vi "Stop task.vi"(8 "error in":errorcluster, 10 "Task list":T1(ring), 11 "Module ID":i32=-1) -> (0 "error out":errorcluster)   [LabVIEW 2020, in "NI DAQ.lvlib"]
doc: "Request to stop all channels within the local task.\n_____\nCreated using DQMH Event Scripter 6.1.0.128."
uses:
  NI DAQ.lvlib
  Stop task Argument--cluster.ctl
  Support/Task list.ctl
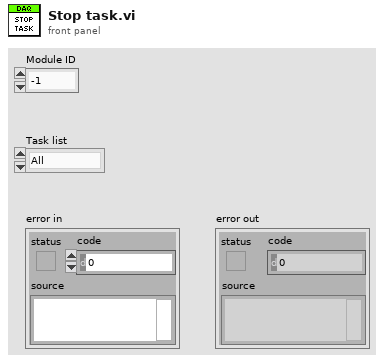
[diagram p1: front panel]
types:
  T1 = enum16{"All", "DO task", "DI task", "AO task", "AI task"}
  T2 = typedef "NI DAQ.lvlib/Stop task Argument--cluster.ctl" = cluster{"Module ID":i32, "Task list":T3}
  T3 = typedef "NI DAQ.lvlib/Task list.ctl" = enum16{"All", "DO task", "DI task", "AO task", "AI task"}
  T4 = typedef "NI DAQ.lvlib/Request Events--cluster.ctl" = cluster{"Stop Module":refnum<user-event>, "Show Panel":refnum<user-event>, "Hide Panel":refnum<user-event>, "Show Diagram":refnum<user-event>, "Get Module Execution Status":refnum<user-event>, "Set device ID":refnum<user-event>, "Get channel list":refnum<user-event>, "Create DO task":refnum<user-event>, "Start task":refnum<user-event>, "Stop task":refnum<user-event>, "Write DO":refnum<user-event>, "Create DI channel":refnum<user-event>, "Read DI":refnum<user-event>, "Get task ref":refnum<user-event>, "Wake up HL":refnum<user-event>, "Sleep HL":refnum<user-event>, "Create AI channel":refnum<user-event>, "Read AI":refnum<user-event>, "Create AO channel":refnum<user-event>, "Write AO":refnum<user-event>, "Validate connection":refnum<user-event>, "Start continous acquisition":refnum<user-event>, "Stop continuous acquisition":refnum<user-event>}
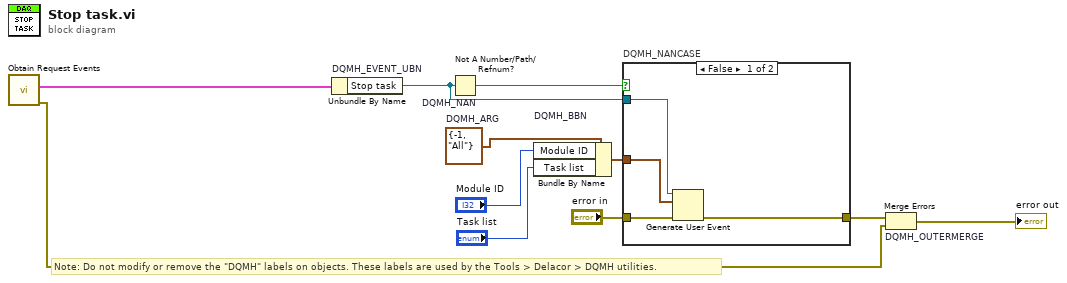
[diagram p0: block diagram]
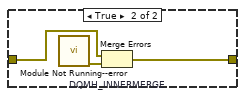
[diagram p2: hidden frame]
diagram:
  w5 = T2 {"Module ID"=-1, "Task list"=enum."All"}  # DQMH_ARG
  # "Note: Do not modify or remove the \"DQMH\" labels on objects. These labels are used by the Tools > Delacor > DQMH utilities."
  n1 = call "Obtain Request Events.vi"() -> ("error out"=w3:errorcluster, "NI DAQ Request Events"=w2:T4)  [unwired: 10 in]
  n2 = Unbundle By Name "DQMH_EVENT_UBN"(w2) -> ("Stop task"=w7:refnum<user-event>)
  n3 = Not A Number/Path/Refnum? "DQMH_NAN"(number/path/refnum=w7) -> (NaN/Path/Refnum?=w8:bool)
  n4 = Bundle By Name "DQMH_BBN"(cluster=w5, "Module ID"="Module ID", "Task list"="Task list") -> (w9:T2)
  n5 = case "DQMH_NANCASE" shown="False" w8 {
    tunnel: "error in" -> [w15 w18]
    tunnel: [w14 w17] -> w6
    tunnel: w7 -> [w13 _]
    tunnel: w9 -> [w12 _]
    frame False {
      n6 = Generate User Event(user event=w13, event data cluster=w12, error in=w15) -> (error out=w14:errorcluster)  [unwired: 1 in, 1 out]
    }
    frame True {
      n7 = call "Module Not Running--error.vi"() -> ("error out"=w16:errorcluster)  [unwired: 11 in]
      n8 = Merge Errors "DQMH_INNERMERGE"(w18, w16) -> (w17:errorcluster)
    }
  }
  n9 = Merge Errors "DQMH_OUTERMERGE"(w6, w3) -> (→"error out":errorcluster)
